vi "Pcre2SubstringFromSubjectByName8 (s).vi"(8 "error in":errorcluster, 9 "Name":string, 10 "Subject":string, 11 "pMatchData":u64 format="%.0x") -> (0 "error out":errorcluster, 2 "Substring":string, 3 "pMatchData":u64 format="%.0x")   [LabVIEW 2021, in "libpcre2-8.lvlib"]
uses:
  libpcre2-8.lvlib
  Pcre2ErrorNull.vi
  Pcre2FnkCallError.vi
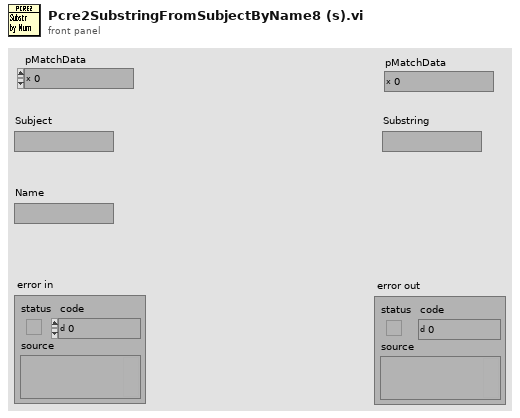
[diagram p1: front panel]
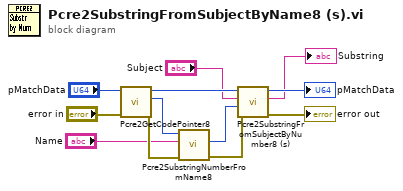
[diagram p0: block diagram]
diagram:
  n1 = call "Pcre2GetCodePointer8.vi"("error in"="error in", "pMatchData"="pMatchData") -> ("error out"=w11:errorcluster, "pCode"=w12:u64, "pMatchData"=w7:u64)  [unwired: 7 in]
  n2 = call "Pcre2SubstringNumberFromName8.vi"("error in"=w11, "Name"="Name", "pCode"=w12) -> ("error out"=w5:errorcluster, "Number"=w4:i32)  [unwired: 6 in, 1 out]
  n3 = call "Pcre2SubstringFromSubjectByNumber8 (s).vi"("error in"=w5, "Number"=w4, "Subject"="Subject", "pMatchData"=w7) -> ("error out"=→"error out":errorcluster, "Substring"=→"Substring":string, "pMatchData"=→"pMatchData":u64)  [unwired: 5 in]
